vi "Get File MD5 Checksum.vi"(8 "error in":errorcluster, 11 "path":path) -> (0 "error out":errorcluster, 3 "MD5":string)   [LabVIEW 2020, in "AIM MIL-STD 1553 Shared.lvlib"]
uses:
  NationalInstruments.VeriStand.Internal
  AIM MIL-STD 1553 Shared.lvlib
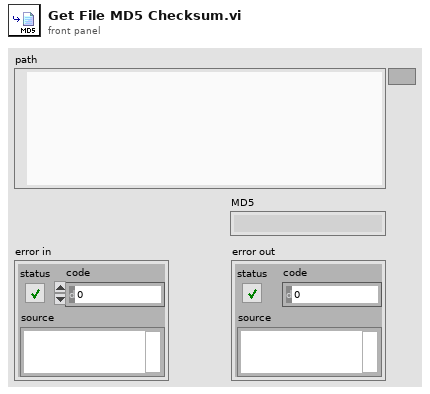
[diagram p1: front panel]
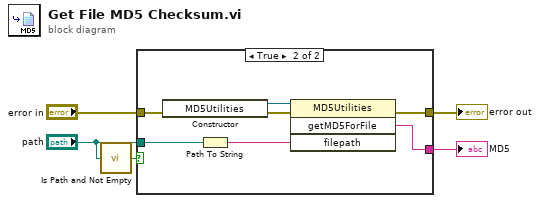
[diagram p0: block diagram]
diagram:
  n1 = call <vilib>:"Is Path and Not Empty.vi"("path"="path") -> ("Is Path and Not Empty?"=w1:bool)  [unwired: 4 in]
  n2 = case shown="True" w1 {
    tunnel: "error in" -> [w6 w10]
    tunnel: "path" -> [_ w9]
    tunnel: [w6 w8] -> w3
    tunnel: [_ w7] -> w2
    frame False {
      # "don't error on empty file path"
    }
    frame True {
      n3 = constructor class="MD5Utilities"(error in=w10) -> (reference out=w11:refnum<k24>, error out=w12:errorcluster)  [unwired: 2 in, 1 out]
      n4 = Path To String(path=w9) -> (string=w13:string)
      n5 = invoke class="MD5Utilities" method="getMD5ForFile"(reference=w11, error in=w12, "filepath"=w13) -> (error out=w8:errorcluster, "getMD5ForFile"=w7:string)  [unwired: 1 in, 2 out]
    }
  }
  "error out" <- w3
  "MD5" <- w2
